vi "SGUI Register Controls.vi"(0 "VI reference (empty)":refnum<vi>, 2 "error in":errorcluster, 6 "control references (empty)":refnum<vi>[](array[refnum]), 8 "register mode (overwrite)":T1=enum."Overwrite", 10 "controls ID (empty)":string) -> (12 "assigned ID":string, 14 "registered control references out":refnum<vi>[](array[refnum]), 16 "error out":errorcluster)   [LabVIEW 2013, in "varilib.lvlib"]
doc: "This VI registers controls for the SGUI library. The registered controls can be then accessed by name instead of reference. All 'access by label' style VIs from the SGUI are made so they will lookup in the stack of the registered controls which is located in global variable. If there are multiple controls with the same name the priority has the last one registered. But all the VIs will lookop through entire stack, not just last assigned batch.\n\nThe function have several options: (i) List of references to controls can be entered directly; (ii) Reference to the VI can be entered in which case this VI will register all available controls on the front panel; (iii) If no control list and no VI reference is assigned this VI will make a list of controls from the calling VI front panel automatically.\n\nWhen 'add to stack' mode is selected the newly found references to controls are added to stack to already available ones. This may be useful when new user panel/dialog is opened and the SGUI shall be used with new controls on this panel. Calling this VI with 'remove last' parameter will remove last registered batch of controls. This can be called for instance when work with subpanel is done. Next option is 'overwrite' which will discard all assigned controls in the stack. This option should be used in the main VI or wherever the controls are registered for the first time in whole application! Final option is 'Remove ID'. It will look for the given ID in the list and removes it if found. Otherwise it returns error.\n\nThis VI ignores input error and will not generate error."
uses:
  varilib.lvlib
  SGUI Assign References Mode.ctl
  SGUI Global Var.vi
  <vilib>/Utility/error.llb/Error Cluster From Error Code.vi
  <vilib>/ErrorRing/Error Ring.xnode
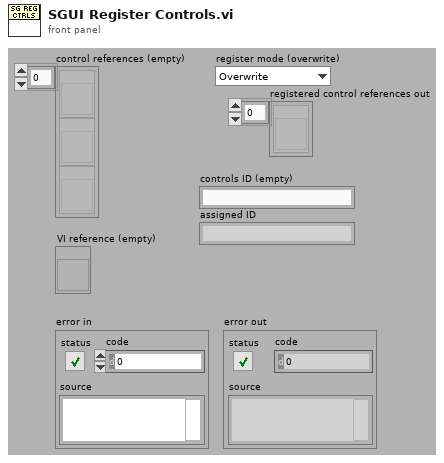
[diagram p1: front panel]
types:
  T1 = typedef "varilib.lvlib/SGUI Assign References Mode.ctl" = enum16{"Add to stack", "Overwrite", "Release last", "Release ID"}
  T2 = cluster{"control references (empty)":refnum<vi>[], string[], "controls ID (empty)":string}
  T3 = cluster{"ctrl refs":refnum<vi>[], "labels":string[], "id":string}[]
  T4 = cluster{"control references (empty)":refnum<vi>[], string[], "controls ID (empty)":string}[]
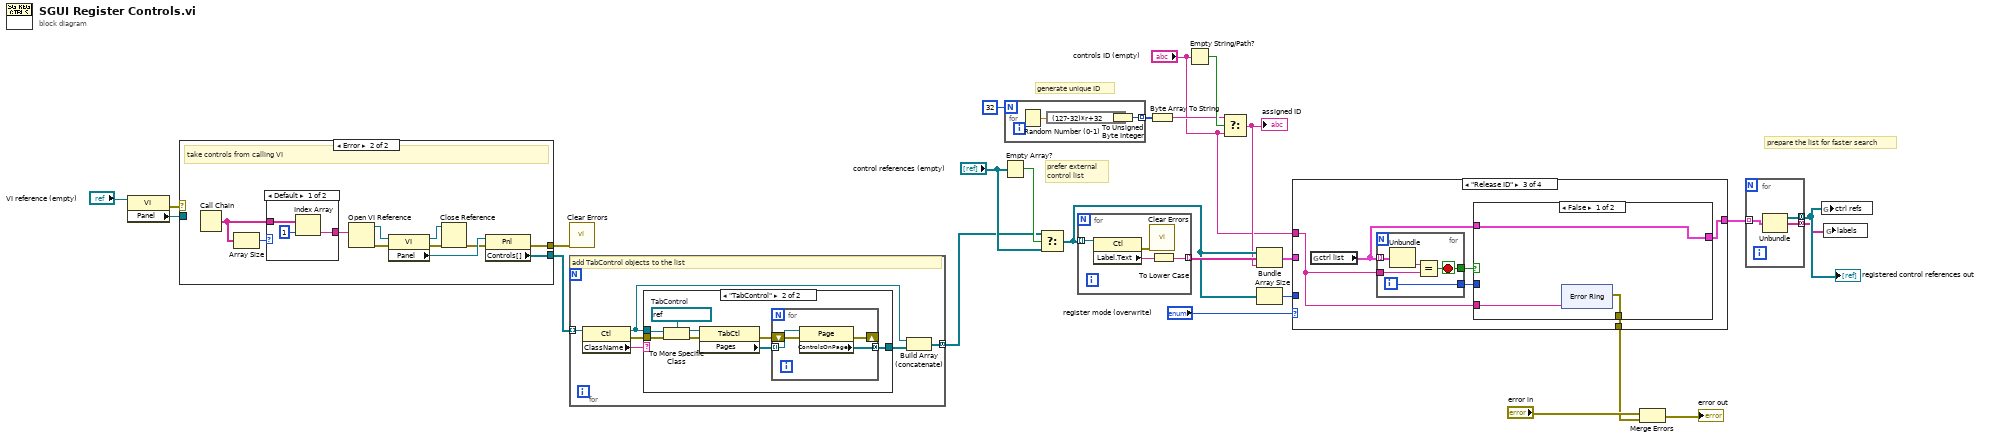
[diagram p0: block diagram]
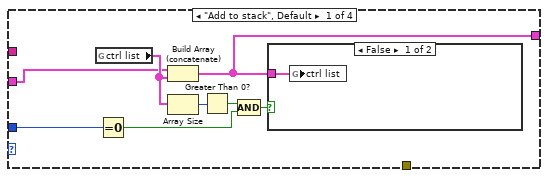
[diagram p3: hidden frame]
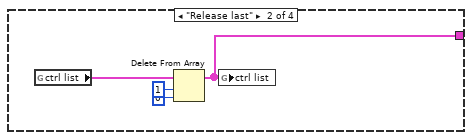
[diagram p5: hidden frame]
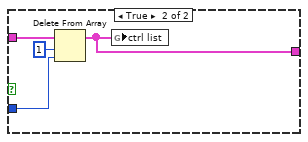
[diagram p6: hidden frame]
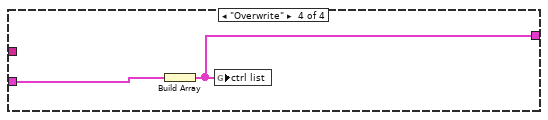
[diagram p7: hidden frame]
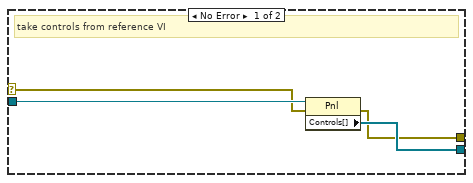
[diagram p8: hidden frame]
diagram:
  # "generate unique ID"
  # "prepare the list for faster search"
  # "prefer external\ncontrol list"
  n1 = property class="VI"(reference="VI reference (empty)") -> (error out=w23:errorcluster, "Panel"=w24:refnum<vi>)  [unwired: 1 in, 1 out]
  n2 = case shown="Error" w23 {
    selector: w23 -> [w26 _]
    tunnel: w24 -> [w29 _]
    tunnel: [w27 w34] -> w20
    tunnel: [w28 w33] -> w11
    frame No Error {
      # "take controls from reference VI"
      n3 = property class="Pnl"(reference=w29, error in=w26) -> (error out=w27:errorcluster, "Controls[]"=w28:refnum<vi>[])  [unwired: 1 out]
    }
    frame Error {
      # "take controls from calling VI"
      n4 = Call Chain() -> (call chain=w39:string[])
      n5 = Array Size(array=w39) -> (size(s)=w40:i32)
      n6 = case shown="Default" w40 {
        tunnel: w39 -> [w43 _]
        tunnel: [w41 _] -> w38
        frame Default {
          n7 = Index Array(array=w43, index=1) -> (element=w41:string)
        }
        frame 0, 1 {
        }
      }
      n8 = Open VI Reference(vi path=w38) -> (vi reference=w36:refnum<vi>, error out=w37:errorcluster)  [unwired: 5 in]
      n9 = property class="VI"(reference=w36, error in=w37) -> (reference out=w31:refnum<vi>, error out=w32:errorcluster, "Panel"=w35:refnum<vi>)
      n10 = Close Reference(reference=w31, error in (no error)=w32) -> (error out=w30:errorcluster)
      n11 = property class="Pnl"(reference=w35, error in=w30) -> (error out=w34:errorcluster, "Controls[]"=w33:refnum<vi>[])  [unwired: 1 out]
    }
  }
  n12 = call <vilib>:"Clear Errors.vi"("error in (no error)"=w20) -> ()  [unwired: 6 in, 1 out]
  n13 = for {
    tunnel: w11 -> [w49] mode=indexing
    tunnel: [w44] -> w10 mode=concatenating
    # "add TabControl objects to the list"
    n14 = property class="Ctl"(reference=w49) -> (reference out=w45:refnum<vi>, error out=w47:errorcluster, "ClassName"=w48:string)  [unwired: 1 in]
    n15 = case shown="\"TabControl\"" w48 {
      tunnel: w45 -> [_ w56]
      tunnel: w47 -> [_ w57]
      tunnel: [_ w50] -> w46
      frame "False", Default {
      }
      frame "TabControl" {
        w55 = refnum<vi> refnum  # TabControl
        n16 = To More Specific Class(target class=w55, reference=w56, error in=w57) -> (specific class reference=w53:refnum<vi>, error out=w54:errorcluster)
        n17 = property class="TabCtl"(reference=w53, error in=w54) -> (error out=w51:errorcluster, "Pages"=w52:refnum<vi>[])  [unwired: 1 out]
        n18 = for {
          tunnel: w52 -> [w60] mode=indexing
          shift-right: [w59] -> _
          shift-left: w51 -> [w61]
          tunnel: [w58] -> w50 mode=concatenating
          n19 = property class="Page"(reference=w60, error in=w61) -> (error out=w59:errorcluster, "ControlsOnPage"=w58:refnum<vi>[])  [unwired: 1 out]
        }
      }
    }
    n20 = Build Array (concatenate)(w45, w46) -> (w44:refnum<vi>[])
  }
  n21 = Empty Array?(array="control references (empty)") -> (empty?=w22:bool)
  n22 = for {
    N: 32 -> [_]
    tunnel: [w62] -> w9 mode=indexing
    n23 = Random Number (0-1)() -> (number: 0 to 1=w64:dbl)
    n24 = expression code="(127-32)*r+32"(w64) -> (w63:dbl)
    n25 = To Unsigned Byte Integer(number=w63) -> (unsigned 8bit integer=w62:u8)
  }
  n26 = Select(t=w10, s=w22, f="control references (empty)") -> (s? t:f=w16:refnum<vi>[])
  n27 = for {
    tunnel: w16 -> [w68] mode=indexing
    tunnel: [w65] -> w18 mode=indexing
    n28 = property class="Ctl"(reference=w68) -> (error out=w67:errorcluster, "Label.Text"=w66:string)  [unwired: 1 in, 1 out]
    n29 = call <vilib>:"Clear Errors.vi"("error in (no error)"=w67) -> ()  [unwired: 6 in, 1 out]
    n30 = To Lower Case(string=w66) -> (all lower case string=w65:string)
  }
  n31 = Byte Array To String(unsigned byte array=w9) -> (string=w6:string)
  n32 = Empty String/Path?(string/path="controls ID (empty)") -> (empty?=w7:bool)
  n33 = Select(t=w6, s=w7, f="controls ID (empty)") -> (s? t:f=w5:string)
  "assigned ID" <- w5
  n34 = Bundle("control references (empty)"=w16, w18, "controls ID (empty)"=w5) -> (w17:T2)  [unwired: 1 in]
  n35 = Array Size(array=w16) -> (size(s)=w15:i32)
  n36 = case shown="\"Release ID\"" "register mode (overwrite)" {
    tunnel: w17 -> [w70 _ _ w108]
    tunnel: w15 -> [w76 _ _ _]
    tunnel: [w69 w78 w84 w107] -> w14
    tunnel: "controls ID (empty)" -> [_ _ w83 _]
    tunnel: [_ _ w82 _] -> w2
    frame "Add to stack", Default {
      n37 = global read "SGUI Global Var.vi" "ctrl list"() -> (w71:T3)
      n38 = Equal To 0?(x=w76) -> (x = 0?=w73:bool)
      n39 = Build Array (concatenate)(w70, w71) -> (w69:T3)
      n40 = Array Size(array=w71) -> (size(s)=w75:i32)
      n41 = Greater Than 0?(x=w75) -> (x > 0?=w74:bool)
      n42 = Compound Arithmetic op=AND(w74, w73) -> (w72:bool)
      n43 = case shown="False" w72 {
        tunnel: w69 -> [w77 _]
        frame False {
          n44 = global write "SGUI Global Var.vi" "ctrl list"(w77) -> ()
        }
        frame True {
        }
      }
    }
    frame "Release last" {
      n45 = global read "SGUI Global Var.vi" "ctrl list"() -> (w81:T3)
      n46 = Delete From Array(array=w81, length=1, index=0) -> (array with subset deleted=w78:T3)  [unwired: 1 out]
      n47 = global write "SGUI Global Var.vi" "ctrl list"(w78) -> ()
    }
    frame "Release ID" {
      n48 = global read "SGUI Global Var.vi" "ctrl list"() -> (w85:T3)
      n49 = for {
        tunnel: w85 -> [w106] mode=indexing
        tunnel: w83 -> [w104]
        tunnel: [w103] -> w86
        tunnel: [w102] -> w87
        i -> [w103]
        stop <- w102 stop-if-true
        n50 = Unbundle(w106) -> ("id"=w105:string)  [unwired: 2 out]
        n51 = Equal?(x=w105, y=w104) -> (x = y?=w102:bool)
      }
      n52 = case shown="False" w87 {
        tunnel: w86 -> [_ w99]
        tunnel: w85 -> [w90 w101]
        tunnel: [w90 w98] -> w84
        tunnel: w83 -> [w89 _]
        tunnel: [w88 _] -> w82
        frame False {
          n53 = xnode "Error Ring"("parameter 0"=w89) -> ("error out"=w88:errorcluster)
        }
        frame True {
          n54 = Delete From Array(array=w101, length=1, index=w99) -> (array with subset deleted=w98:T3)  [unwired: 1 out]
          n55 = global write "SGUI Global Var.vi" "ctrl list"(w98) -> ()
        }
      }
    }
    frame "Overwrite" {
      n56 = Build Array(w108) -> (w107:T4)
      n57 = global write "SGUI Global Var.vi" "ctrl list"(w107) -> ()
    }
  }
  n58 = Merge Errors("error in", w2) -> (→"error out":errorcluster)
  n59 = for {
    tunnel: w14 -> [w111] mode=indexing
    tunnel: [w110] -> w13 mode=concatenating
    tunnel: [w109] -> w12 mode=concatenating
    n60 = Unbundle(w111) -> ("control references (empty)"=w110:refnum<vi>[], "labels"=w109:string[])  [unwired: 1 out]
  }
  "registered control references out" <- w13
  n61 = global write "SGUI Global Var.vi" "ctrl refs"(w13) -> ()
  n62 = global write "SGUI Global Var.vi" "labels"(w12) -> ()
